vi "TCP Connect.vi"(8 "error in (no error)":errorcluster, 11 "Function in":refnum<class "Function.lvclass">) -> (0 "error out":errorcluster, 3 "Function out":refnum<class "Function.lvclass">)   [LabVIEW 2016, in "Function Actor.lvlib" / "Function.lvclass"]
uses:
  <userlib>/Common Components/Function Actor/Function.lvclass
  C:/Program Files (x86)/National Instruments/LabVIEW 2016/vi.lib/ActorFramework/Actor/Actor.lvclass
  <userlib>/Common Components/Function Messages/TCP Connect Msg/TCP Connect Msg.lvclass
  C:/Program Files (x86)/National Instruments/LabVIEW 2016/vi.lib/ActorFramework/Message/Message.lvclass
  <vilib>/ActorFramework/Actor/Actor.lvclass/Actor.ctl
  <vilib>/ActorFramework/Message Enqueuer/Message Enqueuer.lvclass/Message Enqueuer.ctl
  <userlib>/Common Components/Function Actor/Function.lvclass/Function.ctl
  <vilib>/ActorFramework/Message Enqueuer/Init from Existing Queue.vi
  <vilib>/ActorFramework/Message Enqueuer/Message Enqueuer.lvclass
  <vilib>/ActorFramework/Actor/Actor.lvclass
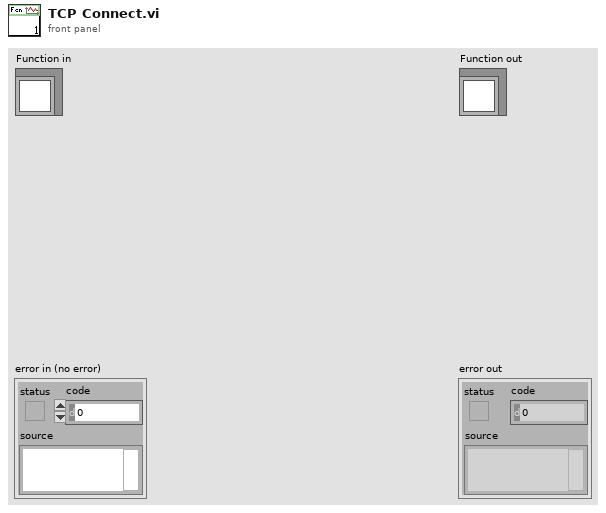
[diagram p1: front panel]
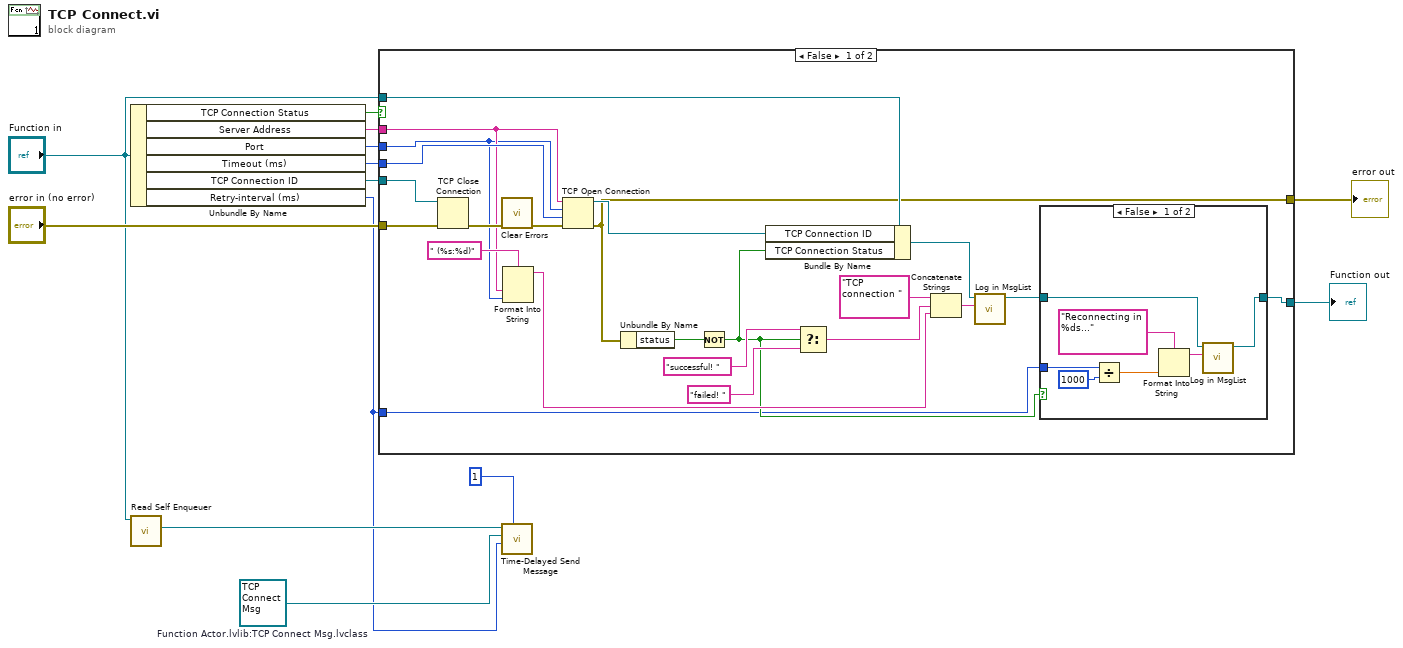
[diagram p0: block diagram]
diagram:
  w2 = refnum<class "TCP Connect Msg.lvclass"> refnum  # Function Actor.lvlib:TCP Connect Msg.lvclass
  n1 = Unbundle By Name("Function in") -> ("TCP Connection Status"=w6:bool, "Server Address"=w9:string, "Port"=w8:u16, "Timeout (ms)"=w13:i32, "TCP Connection ID"=w11:refnum<k5>, "Retry-interval (ms)"=w1:i32)
  n2 = call <vilib>:"Read Self Enqueuer.vi"("Actor"="Function in") -> ("Self Enqueuer"=w4:refnum<class "Message Enqueuer.lvclass">)  [unwired: 10 in]
  n3 = case shown="False" w6 {
    tunnel: "Function in" -> [w36 w46]
    tunnel: w13 -> [w35 _]
    tunnel: [w32 w45] -> w12
    tunnel: w11 -> [w30 _]
    tunnel: "error in (no error)" -> [w28 w45]
    tunnel: w9 -> [w21 _]
    tunnel: w8 -> [w20 _]
    tunnel: [w15 w46] -> w7
    tunnel: w1 -> [w14 _]
    frame False {
      n4 = TCP Close Connection(connection ID=w30, error in (no error)=w28) -> (error out=w29:errorcluster)  [unwired: 1 in, 1 out]
      n5 = call <vilib>:"Clear Errors.vi"("error in (no error)"=w29) -> ("error out"=w27:errorcluster)  [unwired: 5 in, 1 out]
      n6 = Format Into String(format string=" (%s:%d)", w21, w20) -> (resulting string=w19:string)  [unwired: 2 in, 1 out]
      n7 = TCP Open Connection(address=w21, remote port or service name=w20, timeout ms (60000)=w35, error in (no error)=w27) -> (connection ID=w33:refnum<k5>, error out=w32:errorcluster)  [unwired: 1 in]
      n8 = Unbundle By Name(w32) -> ("status"=w31:bool)
      n9 = Not(x=w31) -> (.not. x?=w17:bool)
      n10 = Bundle By Name(cluster=w36, "TCP Connection ID"=w33, "TCP Connection Status"=w17) -> (w34:refnum<class "Function.lvclass">)
      n11 = Select(t="successful! ", s=w17, f="failed! ") -> (s? t:f=w23:string)
      n12 = Concatenate Strings("TCP connection ", w23, w19) -> (w18:string)
      n13 = call-dynamic "Log in MsgList.vi"("Msg"=w18, "Function in"=w34) -> ("Function out"=w16:refnum<class "Function.lvclass">)  [unwired: 8 in, 1 out]
      n14 = case shown="False" w17 {
        tunnel: w16 -> [w42 w44]
        tunnel: [w43 w44] -> w15
        tunnel: w14 -> [w38 _]
        frame False {
          n15 = Divide(x=w38, y=1000) -> (x/y=w39:dbl)
          n16 = Format Into String(format string="Reconnecting in %ds..." ("Msg"), w39) -> (resulting string=w40:string)  [unwired: 2 in, 1 out]
          n17 = call-dynamic "Log in MsgList.vi"("Msg"=w40, "Function in"=w42) -> ("Function out"=w43:refnum<class "Function.lvclass">)  [unwired: 8 in, 1 out]
        }
        frame True {
        }
      }
    }
    frame True {
    }
  }
  "error out" <- w12
  "Function out" <- w7
  n18 = call <vilib>:"Time-Delayed Send Message.vi"("# Copies (0 = infinite repeat)"=u32 1, "Milliseconds To Wait"=w1, "Message"=w2, "Message Enqueuer"=w4) -> ()  [unwired: 6 in, 2 out]
